vi "DIFFERENT ARRAYS FUNCTION.vi"() -> ()   [LabVIEW 2017]
panel:
  out "min index(es)":i32
  out "min value":i32
  out "max index(es)":i32
  out "max value":i32
  out "interleaved array":i32[](array[numeric])
  out "decimated array 2":i32[](array[numeric])
  out "decimated array":i32[](array[numeric])
  out "array (last n elements first)":i32[](array[numeric])
  out "reversed array":i32[](array[numeric])
  out "Array":i32[](array[numeric])
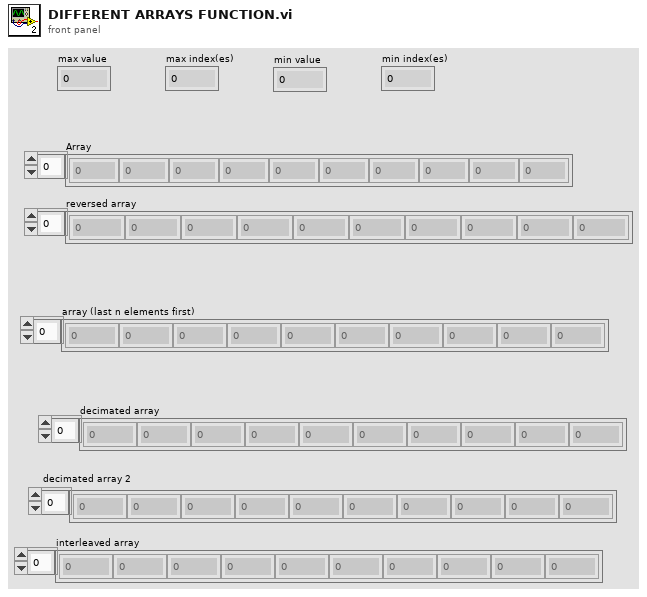
[diagram p1: front panel]
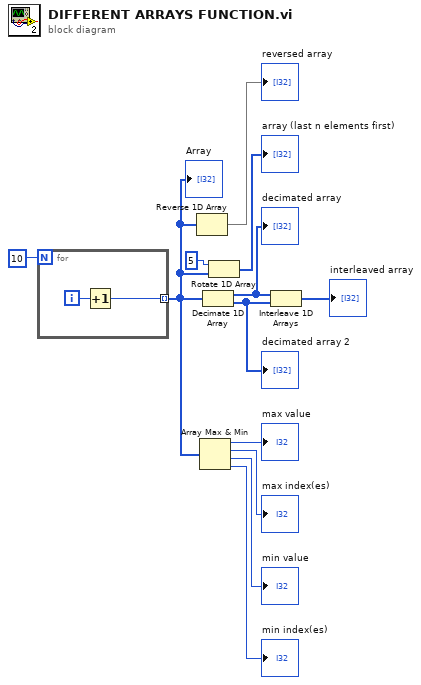
[diagram p0: block diagram]
diagram:
  n1 = for {
    N: 10 -> [_]
    tunnel: [w13] -> w5 mode=indexing
    i -> [w14]
    n2 = Increment(x=w14) -> (x+1=w13:i32)
  }
  "Array" <- w5
  n3 = Reverse 1D Array(array=w5) -> (reversed array=→"reversed array":i32[])
  n4 = Array Max & Min(array=w5) -> (max value=→"max value":i32, max index (indices)=→"max index(es)":i32, min value=→"min value":i32, min index (indices)=→"min index(es)":i32)
  n5 = Decimate 1D Array(w5) -> (w7:i32[], w8:i32[])
  "decimated array" <- w7
  "decimated array 2" <- w8
  n6 = Rotate 1D Array(1:w5, 2:5 ("n")) -> (0:→"array (last n elements first)":i32[])
  n7 = Interleave 1D Arrays(w7, w8) -> (→"interleaved array":i32[])
